vi "Is Done.vi"(8 "error in (no error)":errorcluster, 11 "Monkey in":refnum<class "Monkey.lvclass">) -> (0 "error out":errorcluster, 2 "Is Done?":bool, 3 "Monkey out":refnum<class "Monkey.lvclass">)   [LabVIEW 2022 SP3, in "AoC22.lvlib" / "Monkey.lvclass"]
uses:
  Monkey.lvclass
  Monkey.lvclass/Monkey.ctl
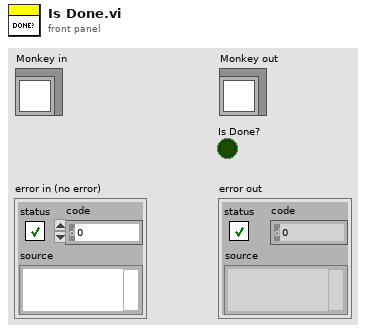
[diagram p1: front panel]
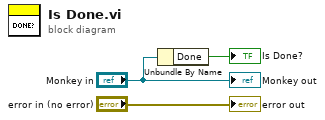
[diagram p0: block diagram]
diagram:
  n1 = Unbundle By Name("Monkey in") -> ("Done"=→"Is Done?":bool)
  "error out" <- "error in (no error)"
  "Monkey out" <- "Monkey in"
